vi "Self-Test.vi"(8 "error in (no error)":errorcluster, 11 "VISA resource name":refnum<visa-resource-name>) -> (0 "error out":errorcluster, 1 "Self-Test Result Message":string, 2 "Last -Test Failed":dbl, 3 "VISA resource name out":refnum<visa-resource-name>)   [LabVIEW 2014, in "Andeen-Hagerling 2700.lvlib"]
doc: "Runs the instrument's self-test routine and returns the test results."
uses:
  Andeen-Hagerling 2700.lvlib
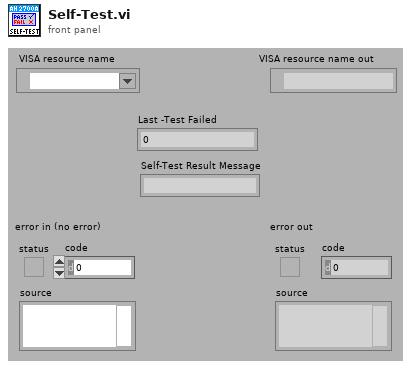
[diagram p1: front panel]
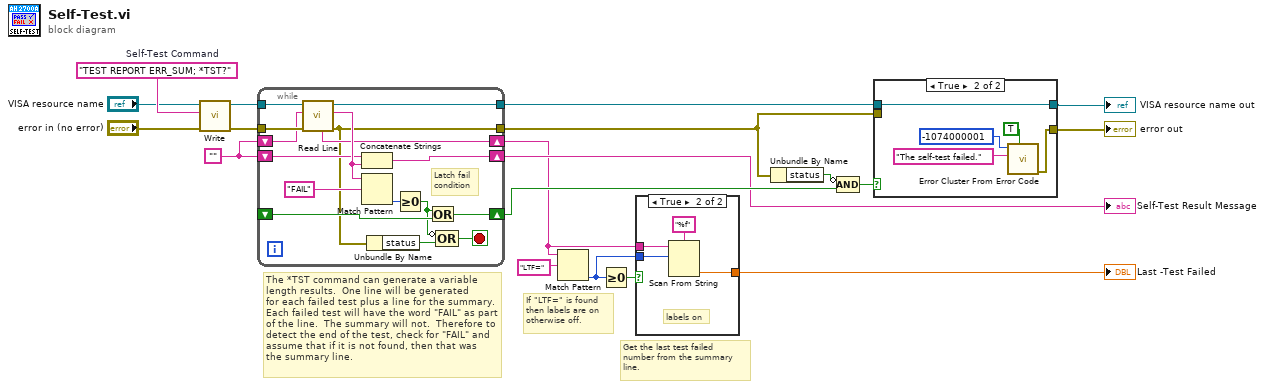
[diagram p0: block diagram]
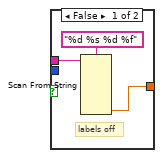
[diagram p2: hidden frame]
diagram:
  w10 = ""
  w15 = "TEST REPORT ERR_SUM; *TST?"  # Self-Test Command
  # "If \"LTF=\" is found\nthen labels are on\notherwise off."
  # "Get the last test failed\nnumber from the summary\nline."
  # "The *TST command can generate a variable\nlength results.  One line will be generated\nfor each failed test plus a line for the summary.\nEach failed test will have the word \"FAIL\" as part\nof the line.  The summary will not.  Therefore to\ndetect the end of the test, check for \"FAIL\" and\nassume that if it is not found, then that was\nthe summary line."
  n1 = call "Write.vi"("error in"="error in (no error)", "command"=w15, "VISA resource name"="VISA resource name") -> ("error out"=w11:errorcluster, "VISA resource name out"=w12:refnum<visa-resource-name>)  [unwired: 7 in]
  n2 = while {
    shift-right: [w25] -> w2
    shift-left: w10 -> [w24]
    tunnel: w12 -> [w28]
    tunnel: w11 -> [w27]
    tunnel: [w29] -> w9
    tunnel: [w23] -> w8
    shift-right: [w30] -> w6
    shift-left: w10 -> [w26]
    shift-right: [w32] -> w7
    shift-left: _ -> [w31]
    stop <- w21 stop-if-true
    # "Latch fail\ncondition"
    n3 = call "Read Line.vi"("error in"=w27, "Previous"=w24, "VISA resource name"=w28) -> ("error out"=w23:errorcluster, "Message"=w35:string, "VISA resource name out"=w29:refnum<visa-resource-name>, "Remaining"=w25:string)  [unwired: 4 in, 1 out]
    n4 = Concatenate Strings(w26, w35) -> (w30:string)
    n5 = Match Pattern(string=w35, regular expression="FAIL") -> (offset past match=w34:i32)  [unwired: 1 in, 3 out]
    n6 = Unbundle By Name(w23) -> ("status"=w22:bool)
    n7 = Greater Or Equal To 0?(x=w34) -> (x >= 0?=w20:bool)
    n8 = Or(x=w20, y=w31) -> (x .or. y?=w32:bool)
    n9 = Compound Arithmetic op=OR(invert w20, w22) -> (w21:bool)
  }
  "Self-Test Result Message" <- w6
  n10 = Match Pattern(string=w2, regular expression="LTF=") -> (offset past match=w3:i32)  [unwired: 1 in, 3 out]
  n11 = Greater Or Equal To 0?(x=w3) -> (x >= 0?=w4:bool)
  n12 = case shown="True" w4 {
    tunnel: w3 -> [_ w41]
    tunnel: [w36 w40] -> w1
    tunnel: w2 -> [w37 w39]
    frame False {
      # "labels off"
      n13 = Scan From String(format string="%d %s %d %f", input string=w37) -> (output 4=w36:dbl)  [unwired: 9 in, 3 out]
    }
    frame True {
      # "labels on"
      n14 = Scan From String(format string="%f", input string=w39, initial scan location=w41) -> (output 1=w40:dbl)  [unwired: 2 in, 3 out]
    }
  }
  "Last -Test Failed" <- w1
  n15 = Unbundle By Name(w8) -> ("status"=w19:bool)
  n16 = Compound Arithmetic op=AND(invert w19, w7) -> (w18:bool)
  n17 = case shown="True" w18 {
    tunnel: w9 -> [w44 w49]
    tunnel: w8 -> [w43 _]
    tunnel: [w43 w45] -> w16
    tunnel: [w44 w49] -> w17
    frame False {
    }
    frame True {
      n18 = call <vilib>:"Error Cluster From Error Code.vi"("show call chain? (False)"=TRUE, "error message (\"\")"="The self-test failed." ("Source (VI Name)"), "error code (0)"=-1074000001 ("Code")) -> ("error out"=w45:errorcluster)  [unwired: 6 in]
    }
  }
  "VISA resource name out" <- w17
  "error out" <- w16
